vi "Read YB.vi"(11 "HE_state in":refnum<class "HE_state_v2.lvclass">) -> (2 "YB":bool[](array[boolean]), 3 "HE_state out":refnum<class "HE_state_v2.lvclass">)   [LabVIEW 2019, in "Heating.lvlib" / "HE_state_v2.lvclass"]
uses:
  HE_state_v2.lvclass
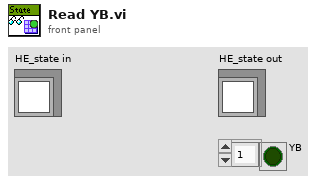
[diagram p1: front panel]
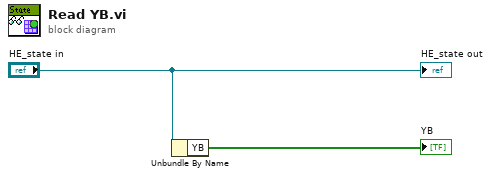
[diagram p0: block diagram]
diagram:
  n1 = Unbundle By Name("HE_state in") -> ("YB"=→"YB":bool[])
  "HE_state out" <- "HE_state in"
